vi "setup excel worksheet.vi"(0 "Last Occupied cell Name reference":refnum<vi>, 1 "Row Max Value Reference":refnum<vi>, 2 "Current Sample Sheet Reference":refnum<vi>, 3 "template file path":path=path "C:/Cascade/templates/Groundwater Profiling Log_empty_labview_template.xlsx", 4 "Excel report file path":path=path "C:/Cascade/Data/Excel Reports/Groundwater Profiling Log_ara1.xlsx", 5 "error in (no error)":errorcluster, 6 "Header path":path=path "C:/Cascade/templates/Fields for Excel sheets.xlsx", 7 "Open Excel Files":bool) -> (8 "subarray":string[][](array[string]), 10 "column max value":i32, 11 "row max value":i32, 12 "Column of Volume":i32, 13 "Worksheet Names":string[](array[string]), 14 "NI_report out":refnum<class "NI_report.lvclass">, 15 "Columns":i32[](array[numeric]), 17 "Number of Sample Sheets":i32, 18 "Select Worksheet Index":i32, 19 "error out":errorcluster)   [LabVIEW 2016]
uses:
  <vilib>/Utility/NIReport.llb/NI_report.lvclass
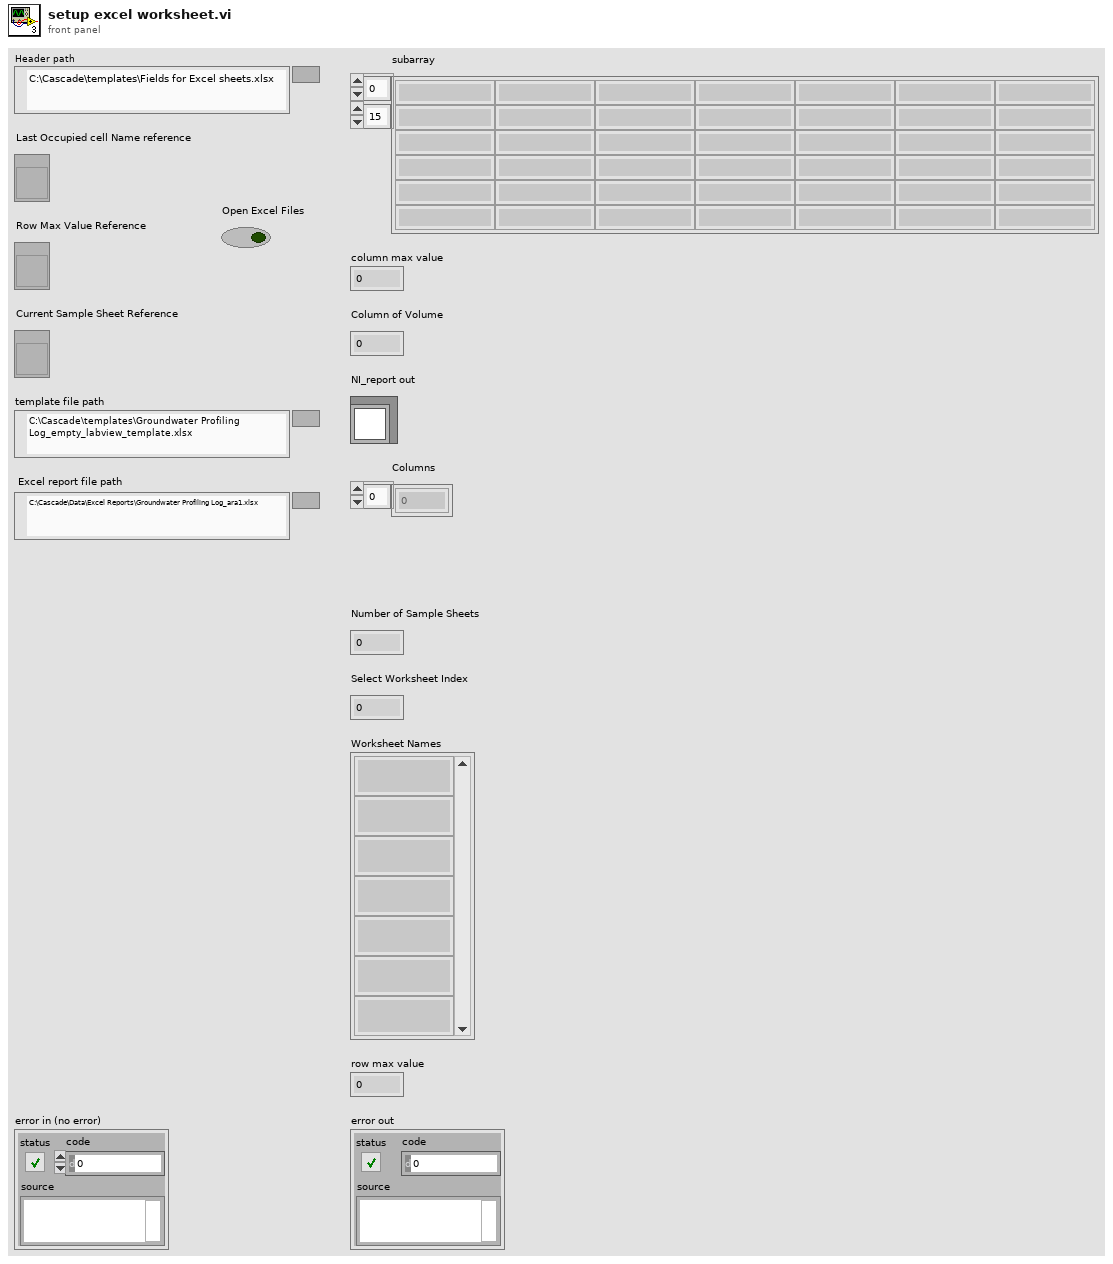
[diagram p1: front panel]
types:
  T1 = enum16{"maximized", "minimized", "normal", "no change"}
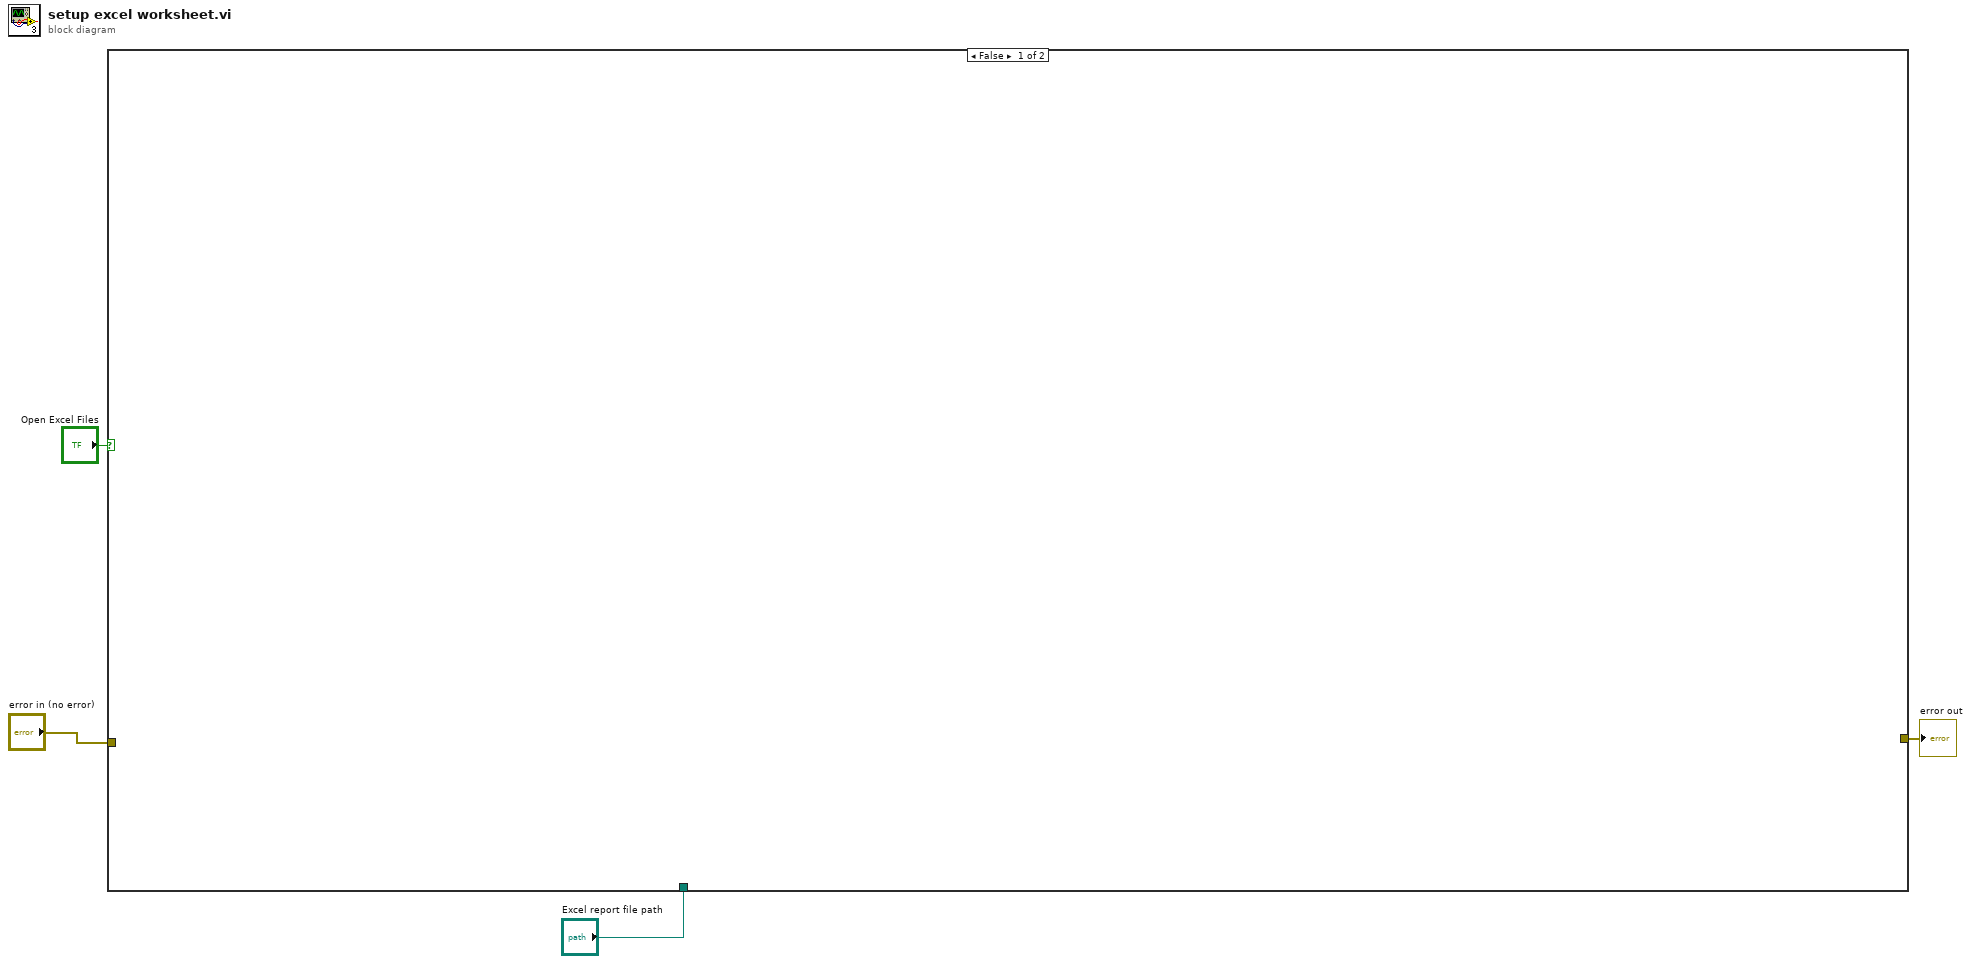
[diagram p0: block diagram]
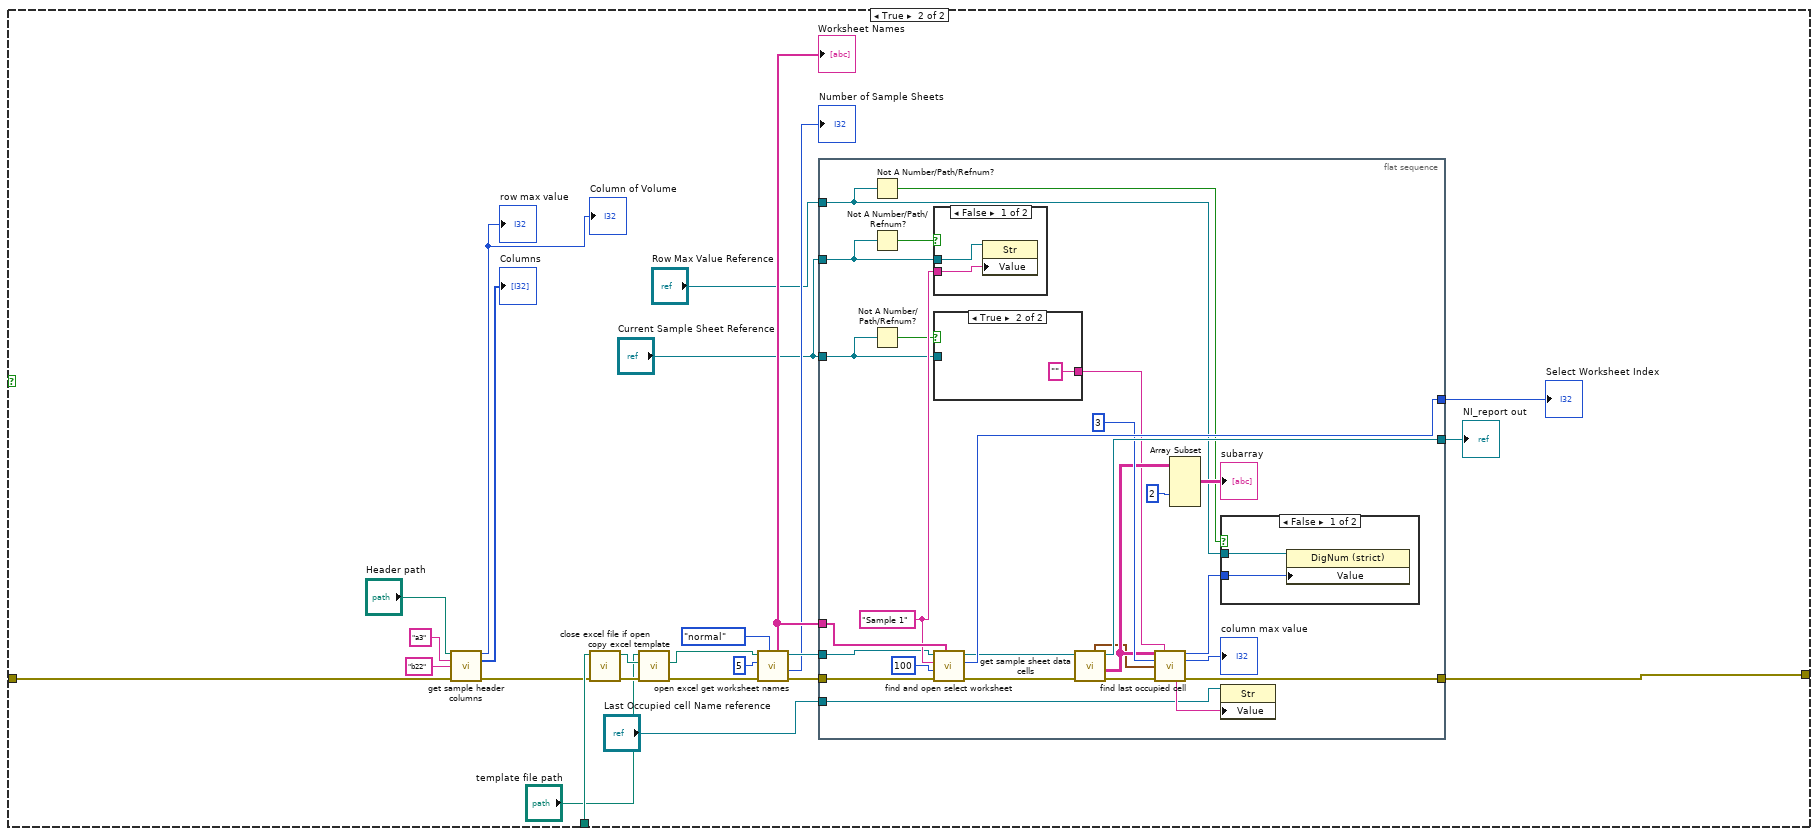
[diagram p2: hidden frame]
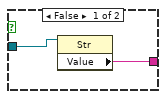
[diagram p4: hidden frame]
diagram:
  n1 = case shown="False" "Open Excel Files" {
    tunnel: [_ w21] -> w4
    tunnel: "Excel report file path" -> [_ w17]
    tunnel: "error in (no error)" -> [_ w5]
    frame False {
    }
    frame True {
      n2 = call "get sample header columns.vi"("report file path"="Header path", "Start Cell Name"="a3", "Stop Cell name"="b22", "error in (no error)"=w5) -> ("Column of Volume"=→"row max value" →"Column of Volume":i32, "Columns"=→"Columns":i32[], "error out"=w9:errorcluster)  [unwired: 2 in, 7 out]
      n3 = call "close excel file if open.vi"("error in (no error)"=w9, "report file path in"=w17) -> ("error out"=w14:errorcluster, "report file path out"=w22:path)  [unwired: 8 in]
      n4 = call "copy excel template.vi"("error in (no error)"=w14, "report file path in"=w22, "template file path in"="template file path") -> ("error out"=w13:errorcluster, "report file path out"=w11:path)  [unwired: 7 in]
      n5 = call "open excel get worksheet names.vi"("window state (normal)"=T1."normal", "error in (no error)"=w13, "milliseconds to wait"=u32 5, "report file path"=w11) -> ("error out"=w25:errorcluster, "Number of Sample Sheets"=→"Number of Sample Sheets":i32, "NI_report out"=w24:refnum<class "NI_report.lvclass">, "Worksheet Names"=w18:string[])  [unwired: 2 in, 2 out]
      "Worksheet Names" <- w18
      n6 = flat-sequence {
        tunnel: w18 -> [w55]
        tunnel: [w53] -> w19
        tunnel: [w51] -> w20
        tunnel: [w49] -> w21
        tunnel: w24 -> [w48]
        tunnel: w25 -> [w47]
        tunnel: "Current Sample Sheet Reference" -> [w31]
        tunnel: "Row Max Value Reference" -> [w35]
        tunnel: "Last Occupied cell Name reference" -> [w36]
        tunnel: "Current Sample Sheet Reference" -> [w33]
        frame #0 {
          w54 = "Sample 1" ("Worksheet Name in")
          n7 = Not A Number/Path/Refnum?(number/path/refnum=w35) -> (NaN/Path/Refnum?=w34:bool)
          n8 = Not A Number/Path/Refnum?(number/path/refnum=w31) -> (NaN/Path/Refnum?=w30:bool)
          n9 = Not A Number/Path/Refnum?(number/path/refnum=w33) -> (NaN/Path/Refnum?=w32:bool)
          n10 = case shown="False" w30 {
            tunnel: w54 -> [w58 _]
            tunnel: w31 -> [w57 _]
            frame False {
              n11 = property class="Str"(reference=w57, "Value"=w58) -> ()  [unwired: 1 in, 2 out]
            }
            frame True {
            }
          }
          n12 = case shown="True" w32 {
            tunnel: [w60 "" ("Value")] -> w40
            tunnel: w33 -> [w59 _]
            frame False {
              n13 = property class="Str"(reference=w59) -> ("Value"=w60:string)  [unwired: 1 in, 2 out]
            }
            frame True {
            }
          }
          n14 = call "find and open select worksheet.vi"("Worksheet Names"=w55, "error in (no error)"=w47, "milliseconds to wait"=u32 100, "Worksheet Name in"=w54, "NI_report in"=w48) -> ("error out"=w50:errorcluster, "Select Worksheet Index"=w53:i32, "NI_report out"=w52:refnum<class "NI_report.lvclass">)  [unwired: 4 in]
          n15 = call "get sample sheet data cells.vi"("error in (no error)"=w50, "NI_report in"=w52) -> ("error out"=w43:errorcluster, "data"=w44:string[][], "NI_report out"=w51:refnum<class "NI_report.lvclass">, "left edge output cluster"=w42:cluster{"row":i32, "column":i32})  [unwired: 5 in, 1 out]
          n16 = call "find last occupied cell.vi"("data"=w44, "Active Sheet"=w40, "Header Rows to remove"=3, "sub array start"=w42, "error in (no error)"=w43) -> ("row max value"=w41:i32, "column max value"=→"column max value":i32, "start of last occupied row"=w39:string, "error out"=w49:errorcluster)  [unwired: 4 in, 3 out]
          n17 = Array Subset(array=w44, index (col)=2 ("index")) -> (→"subarray":string[][])  [unwired: 3 in]
          n18 = case shown="False" w34 {
            tunnel: w41 -> [w63 _]
            tunnel: w35 -> [w62 _]
            frame False {
              n19 = property class="DigNum (strict)"(reference=w62, "Value"=w63) -> ()  [unwired: 1 in, 2 out]
            }
            frame True {
            }
          }
          n20 = property class="Str"(reference=w36, "Value"=w39) -> ()  [unwired: 1 in, 2 out]
        }
      }
      "NI_report out" <- w20
      "Select Worksheet Index" <- w19
    }
  }
  "error out" <- w4
